vi "Add Glyph to Icon.vi"(8 "error in (no error)":errorcluster, 10 "Glyph Path":path, 11 "Control Path":path) -> (0 "error out":errorcluster)   [LabVIEW 2023, in "VILab.lvlib"]
uses:
  <vilib>/Utility/miscctls.llb/LVPoint32TypeDef.ctl
  <vilib>/LabVIEW Icon API/API_User Layer Data.ctl
  <vilib>/picture/picture.llb/imagedata.ctl
  VILab.lvlib
  <vilib>/LabVIEW Icon API/LabVIEW Icon API.lvlib
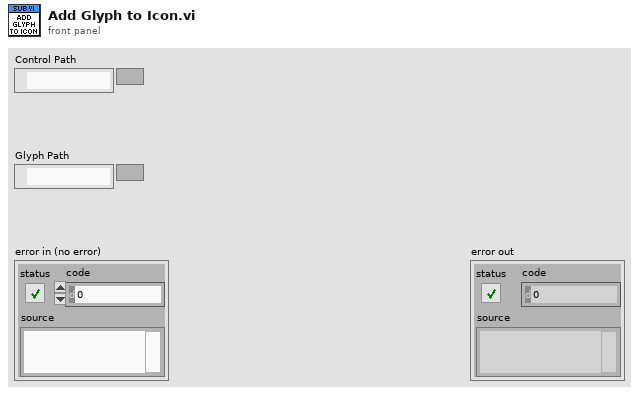
[diagram p1: front panel]
types:
  T1 = typedef "imagedata.ctl" = cluster{"image type":i32, "image depth":i32, "image":u8[], "mask":u8[], "colors":u32[], "Rectangle":cluster{"left":i16, "top":i16, "right":i16, "bottom":i16}}
  T2 = typedef "LVPoint32TypeDef.ctl" = cluster{"Horizontal":i32, "Vertical":i32}
  T3 = typedef "LabVIEW Icon API.lvlib/API_User Layer Data.ctl" = cluster{"Layer name":string, "Origin":T2, "Icon image data":T1}
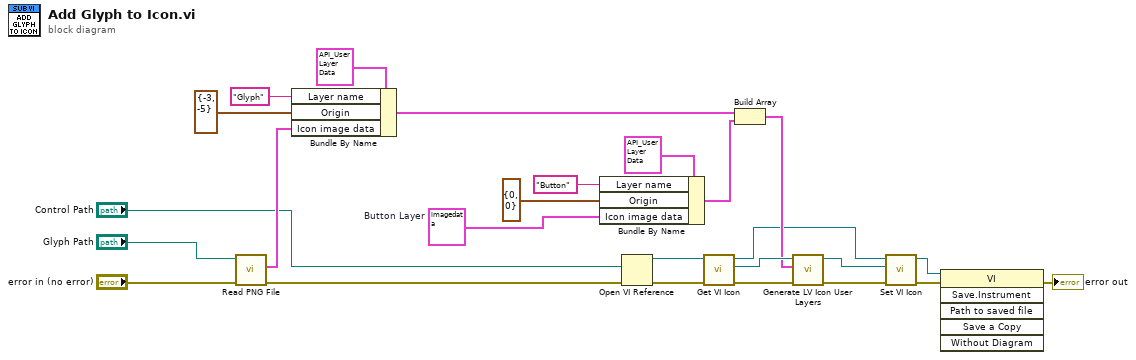
[diagram p0: block diagram]
diagram:
  w6 = T1 {"image type"=0, "image depth"=8, "image"=array[1024 elements], "mask"=[128, 0, 0, 0, 127, 255, 255, 254, 127, 255, 255, 254, 127, 255, 255, 254, 127, 255, 255, 254, 127, 255, 255, 254, 127, 255, 255, 254, 127, 255, 255, 254, 127, 255, 255, 254, 127, 255, 255, 254, 127, 255, 255, 254, 127, 255, 255, 254, 127, 255, 255, 254, 127, 255, 255, 254, 127, 255, 255, 254, 127, 255, 255, 254, 127, 255, 255, 254, 127, 255, 255, 254, 127, 255, 255, 254, 127, 255, 255, 254, 127, 255, 255, 254, 127, 255, 255, 254, 127, 255, 255, 254, 127, 255, 255, 254, 127, 255, 255, 254, 127, 255, 255, 254, 127, 255, 255, 254, 127, 255, 255, 254, 127, 255, 255, 254, 127, 255, 255, 254, 127, 255, 255, 254, 0, 0, 0, 0], "colors"=[16777215, 16777164, 16777113, 16777062, 16777011, 16776960, 16764159, 16764108, 16764057, 16764006, 16763955, 16763904, 16751103, 16751052, 16751001, 16750950, 16750899, 16750848, 16738047, 16737996, 16737945, 16737894, 16737843, 16737792, 16724991, 16724940, 16724889, 16724838, 16724787, 16724736, 16711935, 16711884, 16711833, 16711782, 16711731, 16711680, 13434879, 13434828, 13434777, 13434726, 13434675, 13434624, 13421823, 13421772, 13421721, 13421670, 13421619, 13421568, 13408767, 13408716, 13408665, 13408614, 13408563, 13408512, 13395711, 13395660, 13395609, 13395558, 13395507, 13395456, 13382655, 13382604, 13382553, 13382502, 13382451, 13382400, 13369599, 13369548, 13369497, 13369446, 13369395, 13369344, 10092543, 10092492, 10092441, 10092390, 10092339, 10092288, 10079487, 10079436, 10079385, 10079334, 10079283, 10079232, 10066431, 10066380, 10066329, 10066278, 10066227, 10066176, 10053375, 10053324, 10053273, 10053222, 10053171, 10053120, 10040319, 10040268, 10040217, 10040166, 10040115, 10040064, 10027263, 10027212, 10027161, 10027110, 10027059, 10027008, 6750207, 6750156, 6750105, 6750054, 6750003, 6749952, 6737151, 6737100, 6737049, 6736998, 6736947, 6736896, 6724095, 6724044, 6723993, 6723942, 6723891, 6723840, 6711039, 6710988, 6710937, 6710886, 6710835, 6710784, 6697983, 6697932, 6697881, 6697830, 6697779, 6697728, 6684927, 6684876, 6684825, 6684774, 6684723, 6684672, 3407871, 3407820, 3407769, 3407718, 3407667, 3407616, 3394815, 3394764, 3394713, 3394662, 3394611, 3394560, 3381759, 3381708, 3381657, 3381606, 3381555, 3381504, 3368703, 3368652, 3368601, 3368550, 3368499, 3368448, 3355647, 3355596, 3355545, 3355494, 3355443, 3355392, 3342591, 3342540, 3342489, 3342438, 3342387, 3342336, 65535, 65484, 65433, 65382, 65331, 65280, 52479, 52428, 52377, 52326, 52275, 52224, 39423, 39372, 39321, 39270, 39219, 39168, 26367, 26316, 26265, 26214, 26163, 26112, 13311, 13260, 13209, 13158, 13107, 13056, 255, 204, 153, 102, 51, 15597568, 14483456, 12255232, 11141120, 8912896, 7798784, 5570560, 4456448, 2228224, 1114112, 60928, 56576, 47872, 43520, 34816, 30464, 21760, 17408, 8704, 4352, 238, 221, 187, 170, 136, 119, 85, 68, 34, 17, 15658734, 14540253, 12303291, 11184810, 8947848, 7829367, 5592405, 4473924, 2236962, 1118481, 0], "Rectangle"={"left"=0, "top"=0, "right"=32, "bottom"=32}}  # Button Layer
  n1 = call <vilib>:"Read PNG File.vi"("error in (no error)"="error in (no error)", "path to PNG file"="Glyph Path") -> ("error out"=w4:errorcluster, "image data"=w17:T1)  [unwired: 7 in, 1 out]
  n2 = Bundle By Name(cluster=T3 {"Layer name"="", "Origin"={"Horizontal"=0, "Vertical"=0}, "Icon image data"={"image type"=0, "image depth"=0, "image"=[], "mask"=[], "colors"=[], "Rectangle"={"left"=0, "top"=0, "right"=0, "bottom"=0}}} ("User layer"), "Layer name"="Glyph", "Origin"=T2 {"Horizontal"=-3, "Vertical"=-5}, "Icon image data"=w17) -> (w16:T3)
  n3 = Bundle By Name(cluster=T3 {"Layer name"="", "Origin"={"Horizontal"=0, "Vertical"=0}, "Icon image data"={"image type"=0, "image depth"=0, "image"=[], "mask"=[], "colors"=[], "Rectangle"={"left"=0, "top"=0, "right"=0, "bottom"=0}}} ("User layer"), "Layer name"="Button", "Origin"=T2 {"Horizontal"=0, "Vertical"=0}, "Icon image data"=w6) -> (w15:T3)
  n4 = Open VI Reference(vi path="Control Path", error in (no error)=w4) -> (vi reference=w7:refnum<vi>, error out=w8:errorcluster)  [unwired: 4 in]
  n5 = call <vilib>:"Get VI Icon.vi"("error in (no error)"=w8, "VI Refnum in"=w7) -> ("error out"=w25:errorcluster, "Icon"=w24:refnum<class "Icon.lvclass">, "VI Refnum out"=w10:refnum<vi>)  [unwired: 7 in]
  n6 = Build Array(w16, w15) -> (w11:T3[])
  n7 = call <vilib>:"Generate LV Icon User Layers.vi"("error in (no error)"=w25, "User layers"=w11, "Icon in"=w24) -> ("error out"=w14:errorcluster, "Icon out"=w12:refnum<class "Icon.lvclass">)  [unwired: 7 in]
  n8 = call <vilib>:"Set VI Icon.vi"("error in (no error)"=w14, "Icon"=w12, "VI Refnum in"=w10) -> ("error out"=w13:errorcluster, "VI Refnum out"=w9:refnum<vi>)  [unwired: 7 in]
  n9 = invoke class="VI" method="Save.Instrument"(reference=w9, error in=w13) -> (error out=→"error out":errorcluster)  [unwired: 4 in, 5 out]
